vi "Set_Output_State.vi"(2 "error in":errorcluster, 3 "register 2 (8-13)":bool[](array[boolean])=[FALSE, FALSE, FALSE, FALSE, FALSE, FALSE], 4 "register 1 (2-7)":bool[](array[boolean]), 5 "VISA arduino in":refnum<visa-resource-name>) -> (0 "error out":errorcluster, 1 "VISA arduino out":refnum<visa-resource-name>)   [LabVIEW 2021]
uses:
  <vilib>/Utility/error.llb/Error Cluster From Error Code.vi
  <vilib>/ErrorRing/Error Ring.xnode
panel:
  out "delay":u32
  out "comand 2":string
  out "comand 1":string
  # "Private"
  # "Public"
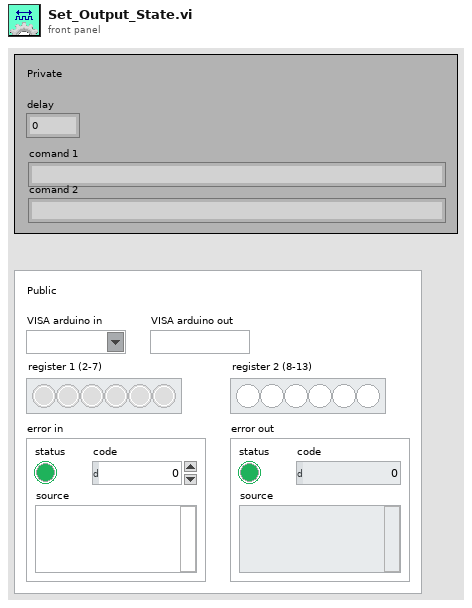
[diagram p1: front panel]
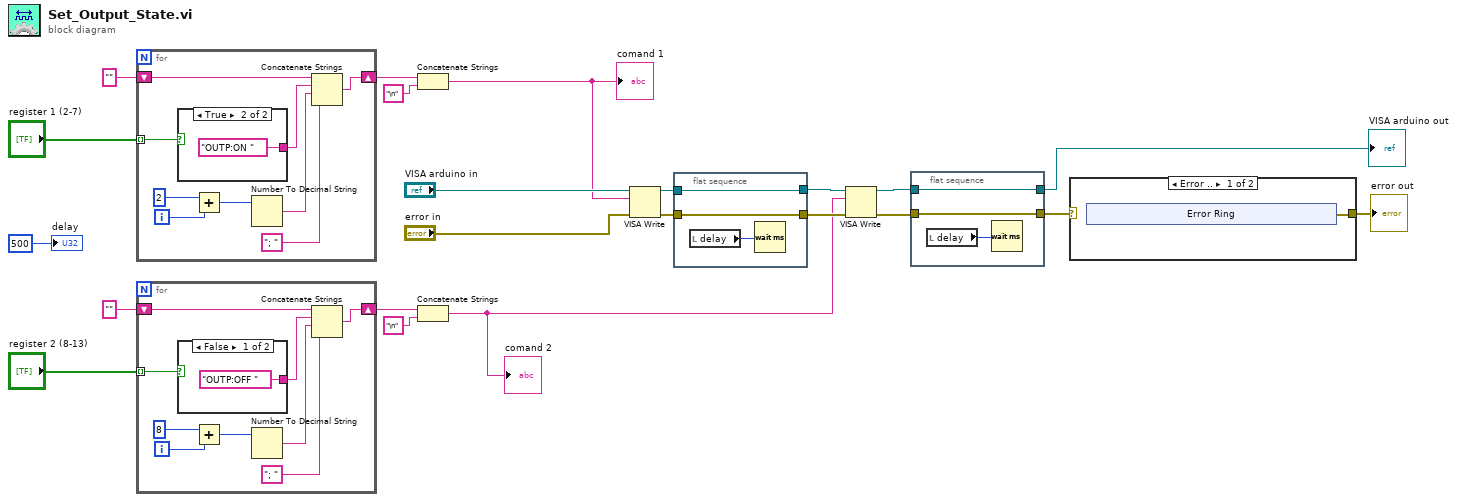
[diagram p0: block diagram]
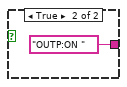
[diagram p3: hidden frame]
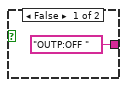
[diagram p4: hidden frame]
diagram:
  n1 = for {
    shift-right: [w27] -> w19
    shift-left: "" -> [w26]
    tunnel: "register 1 (2-7)" -> [w31] mode=indexing
    i -> [w29]
    n2 = case shown="True" w31 {
      tunnel: ["OUTP:OFF " "OUTP:ON "] -> w25
      frame False {
      }
      frame True {
      }
    }
    n3 = Add(x=2, y=w29) -> (x+y=w28:i32)
    n4 = Number To Decimal String(number=w28) -> (decimal integer string=w24:string)  [unwired: 1 in]
    n5 = Concatenate Strings(w26, w25, w24, "; ") -> (w27:string)
  }
  n6 = for {
    shift-right: [w38] -> w18
    shift-left: "" -> [w37]
    tunnel: "register 2 (8-13)" -> [w42] mode=indexing
    i -> [w40]
    n7 = case shown="False" w42 {
      tunnel: ["OUTP:OFF " "OUTP:ON "] -> w36
      frame False {
      }
      frame True {
      }
    }
    n8 = Add(x=8, y=w40) -> (x+y=w39:i32)
    n9 = Number To Decimal String(number=w39) -> (decimal integer string=w35:string)  [unwired: 1 in]
    n10 = Concatenate Strings(w37, w36, w35, "; ") -> (w38:string)
  }
  n11 = Concatenate Strings(w19, "\n" ("string")) -> (w12:string)
  "comand 1" <- w12
  n12 = Concatenate Strings(w18, "\n" ("string")) -> (w7:string)
  "comand 2" <- w7
  n13 = VISA Write(VISA resource name="VISA arduino in", write buffer=w12, error in (no error)="error in") -> (VISA resource name out=w11:refnum<visa-resource-name>, error out=w10:errorcluster)  [unwired: 1 out]
  n14 = flat-sequence {
    tunnel: w11 -> [w46]
    tunnel: w10 -> [w45]
    tunnel: [w46] -> w9
    tunnel: [w45] -> w8
    frame #0 {
      n15 = local read "delay"() -> (w47:u32)
      n16 = Wait (ms)(milliseconds to wait=w47) -> ()  [unwired: 1 out]
    }
  }
  n17 = VISA Write(VISA resource name=w9, write buffer=w7, error in (no error)=w8) -> (VISA resource name out=w6:refnum<visa-resource-name>, error out=w5:errorcluster)  [unwired: 1 out]
  n18 = flat-sequence {
    tunnel: w6 -> [w48]
    tunnel: w5 -> [w49]
    tunnel: [w49] -> w4
    tunnel: [w48] -> w2
    frame #0 {
      n19 = local read "delay"() -> (w50:u32)
      n20 = Wait (ms)(milliseconds to wait=w50) -> ()  [unwired: 1 out]
    }
  }
  n21 = case shown="Error .." w4 {
    selector: w4 -> [_ w57]
    tunnel: [w51 w57] -> w3
    frame Error {
      n22 = xnode "Error Ring"() -> ("error out"=w51:errorcluster)
    }
    frame No Error {
    }
  }
  "error out" <- w3
  "VISA arduino out" <- w2
  "delay" <- u32 500
